vi "Bradford Transformation.vi"(1 "XYZs":dbl[](array[numeric]), 2 "Illuminants":T1) -> (0 "XYZd":dbl[](array[numeric]) format="%.2f")   [LabVIEW 2013]
uses:
  <vilib>/Analysis/baseanly.llb/A x Vector.vi
  <vilib>/Analysis/baseanly.llb/Real A x B.vi
  <vilib>/Analysis/baseanly.llb/Real Inverse Matrix.vi
  <vilib>/Analysis/7linalg.llb/Create Special Real Matrix.vi
  <vilib>/Analysis/NI_AALBase.lvlib
  <vilib>/Analysis/NI_AALPro.lvlib
panel:
  out "WD":dbl[](array[numeric])
  out "WDe":bool
  out "WSe":bool
  out "WS":dbl[](array[numeric])
  out "Breadford Matrix":dbl[][](array[numeric])
  # "Chromatic Adaptation Evaluation"
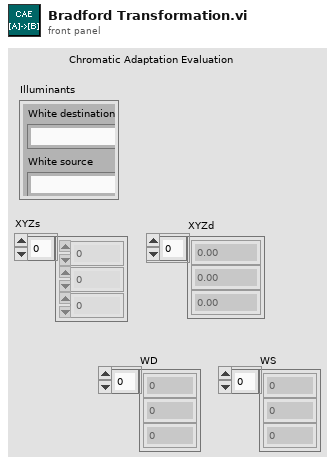
[diagram p1: front panel]
types:
  T1 = cluster{"White destination":string, "White source":string}
  T2 = typedef "NI_Matrix.lvlib/RealMatrix.ctl" = dbl[][]
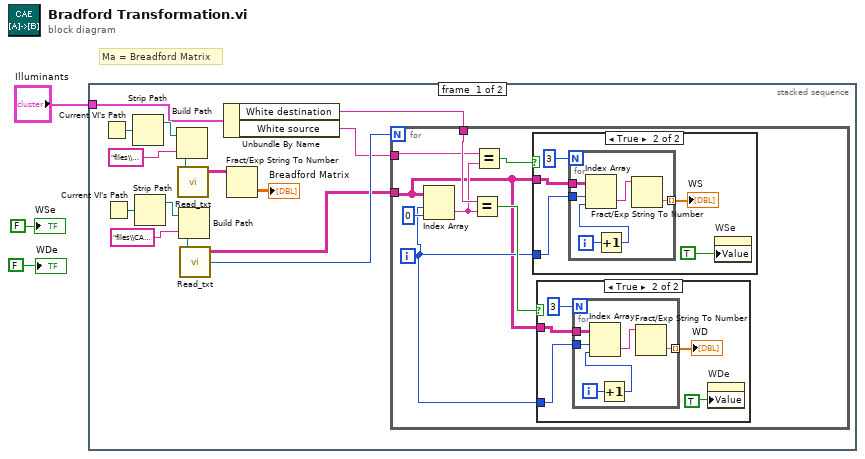
[diagram p0: block diagram]
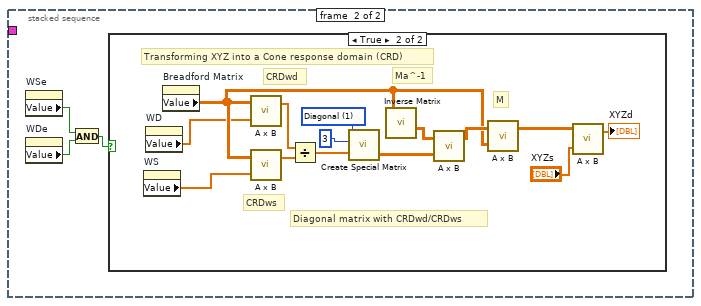
[diagram p4: hidden frame]
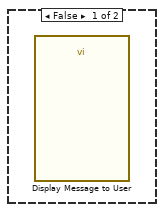
[diagram p5: hidden frame]
diagram:
  # "Ma = Breadford Matrix"
  n1 = stacked-sequence {
    tunnel: "Illuminants" -> [w6 _]
    frame #0 {
      n2 = Current VI's Path() -> (path=w17:path)
      n3 = Current VI's Path() -> (path=w11:path)
      n4 = Strip Path(path=w17) -> (stripped path=w16:path)  [unwired: 1 out]
      n5 = Strip Path(path=w11) -> (stripped path=w10:path)  [unwired: 1 out]
      n6 = Build Path(base path=w16, name or relative path="files\\Bradford.txt") -> (appended path=w15:path)
      n7 = call "Read_txt.vi"("file path (dialog if empty)"=w15) -> ("Elements"=w14:string[][])  [unwired: 2 out]
      n8 = Build Path(base path=w10, name or relative path="files\\CAS.txt") -> (appended path=w9:path)
      n9 = call "Read_txt.vi"("file path (dialog if empty)"=w9) -> ("Elements"=w7:string[][], "Rows"=w8:i32)  [unwired: 1 out]
      n10 = Unbundle By Name(w6) -> ("White destination"=w5:string, "White source"=w4:string)
      n11 = Fract/Exp String To Number(string=w14) -> (number=→"Breadford Matrix":dbl[][])  [unwired: 3 in, 1 out]
      n12 = for {
        N: w8 -> [_]
        tunnel: w7 -> [w19]
        tunnel: w5 -> [w26]
        tunnel: w4 -> [w25]
        i -> [w20]
        n13 = Index Array(array=w19, index (row)=w20, index (col)=0 ("disabled index (col)")) -> (element=w24:string)
        n14 = Equal?(x=w26, y=w24) -> (x = y?=w21:bool)
        n15 = Equal?(x=w25, y=w24) -> (x = y?=w22:bool)
        n16 = case shown="True" w22 {
          tunnel: w19 -> [_ w41]
          tunnel: w20 -> [_ w40]
          frame False {
          }
          frame True {
            n17 = for {
              N: 3 -> [_]
              tunnel: w41 -> [w48]
              tunnel: w40 -> [w47]
              tunnel: [w45] -> w39 mode=indexing
              i -> [w44]
              n18 = Increment(x=w44) -> (x+1=w43:i32)
              n19 = Index Array(array=w48, index (row)=w47, index (col)=w43) -> (element=w46:string)
              n20 = Fract/Exp String To Number(string=w46) -> (number=w45:dbl)  [unwired: 3 in, 1 out]
            }
            "WS" <- w39
            n21 = property on="WSe" class="Bool (strict)"("Value"=TRUE) -> ()  [unwired: 2 in, 2 out]
          }
        }
        n22 = case shown="True" w21 {
          tunnel: w19 -> [_ w30]
          tunnel: w20 -> [_ w29]
          frame False {
          }
          frame True {
            n23 = for {
              N: 3 -> [_]
              tunnel: w30 -> [w37]
              tunnel: w29 -> [w36]
              tunnel: [w34] -> w28 mode=indexing
              i -> [w32]
              n24 = Increment(x=w32) -> (x+1=w33:i32)
              n25 = Index Array(array=w37, index (row)=w36, index (col)=w33) -> (element=w35:string)
              n26 = Fract/Exp String To Number(string=w35) -> (number=w34:dbl)  [unwired: 3 in, 1 out]
            }
            "WD" <- w28
            n27 = property on="WDe" class="Bool (strict)"("Value"=TRUE) -> ()  [unwired: 2 in, 2 out]
          }
        }
      }
    }
    frame #1 {
      n28 = property on="WSe" class="Bool (strict)"() -> ("Value"=w50:bool)  [unwired: 2 in, 2 out]
      n29 = property on="WDe" class="Bool (strict)"() -> ("Value"=w49:bool)  [unwired: 2 in, 2 out]
      n30 = And(x=w50, y=w49) -> (x .and. y?=w51:bool)
      n31 = case shown="True" w51 {
        frame False {
          n32 = call "Display Message to User"() -> ()  [unwired: 10 in, 2 out]
        }
        frame True {
          w62 = 1 items=["Identity", "Diagonal", "Toeplitz", "Vandermonde", "Companion", "Hankel", "Hadamard", "Wilkinson", "Hilbert", "Inverse Hilbert", "Rosser", "Pascal"] ("matrix type")
          # "M"
          # "Diagonal matrix with CRDwd/CRDws"
          # "CRDws"
          # "CRDwd"
          # "Ma^-1"
          # "Transforming XYZ into a Cone response domain (CRD)"
          n33 = property on="WS" class="Arr (strict)"() -> ("Value"=w54:dbl[])  [unwired: 2 in, 2 out]
          n34 = property on="WD" class="Arr (strict)"() -> ("Value"=w53:dbl[])  [unwired: 2 in, 2 out]
          n35 = property on="Breadford Matrix" class="Arr (strict)"() -> ("Value"=w59:dbl[][])  [unwired: 2 in, 2 out]
          n36 = call-poly <vilib>:"A x B.vi"("Vector"=w53, "A"=w59) -> ("A x Vector"=w65:dbl[])  [unwired: 1 out]
          n37 = call-poly <vilib>:"A x B.vi"("Vector"=w54, "A"=w59) -> ("A x Vector"=w64:dbl[])  [unwired: 1 out]
          n38 = Divide(x=w65, y=w64) -> (x/y=w57:dbl[])
          n39 = call-poly <vilib>:"Create Special Matrix.vi"("matrix type"=w62, "matrix size"=3, "Input Vector1"=w57) -> ("Special Matrix"=w61:T2)  [unwired: 2 in, 1 out]
          n40 = call-poly <vilib>:"Inverse Matrix.vi"("Input Matrix"=w59) -> ("Inverse Matrix"=w58:T2)  [unwired: 1 in, 1 out]
          n41 = call-poly <vilib>:"A x B.vi"("B"=w61, "A"=w58) -> ("A x B"=w60:T2)  [unwired: 1 out]
          n42 = call-poly <vilib>:"A x B.vi"("B"=w59, "A"=w60) -> ("A x B"=w56:T2)  [unwired: 1 out]
          n43 = call-poly <vilib>:"A x B.vi"("Vector"="XYZs", "A"=w56) -> ("A x Vector"=→"XYZd":dbl[])  [unwired: 1 out]
        }
      }
    }
  }
  "WSe" <- FALSE ("WSe")
  "WDe" <- FALSE ("WSe")
